vi "Set Pos Ctrl Paras.vi"(8 "error in (no error)":errorcluster, 10 "Pos Ctrl Paras":T1={"Tolerance(deg)"=0.5, "Loop Time(ms)"=10, "Min Frequency(hz)"=40.0} {"Min Frequency(hz)" format="%#_13g"}, 11 "SGDV_Ctrl_Class in":refnum<class "SGDV Motor.lvclass">) -> (0 "error out":errorcluster, 3 "SGDV_Ctrl_Class out":refnum<class "SGDV Motor.lvclass">)   [LabVIEW 2013, in "SGDV_Ctrl_v13_lib.lvlib" / "SGDV Motor.lvclass"]
uses:
  SGDV Motor.lvclass
  Controls and General VIs/Pos Ctrl Paras.ctl
  SGDV Motor.lvclass/SGDV Motor.ctl
  SGDV_Ctrl_v13_lib.lvlib
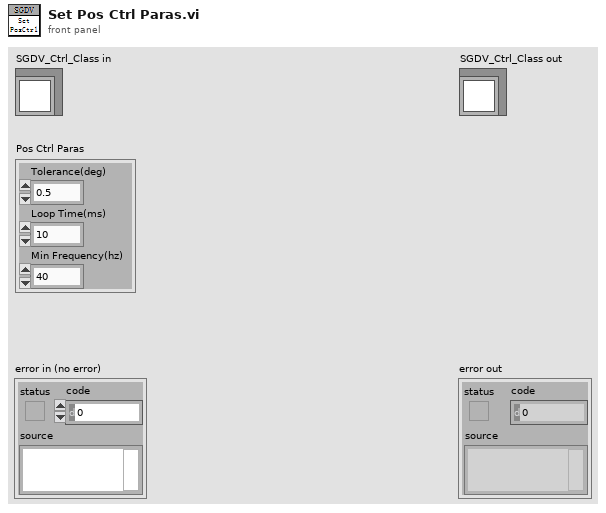
[diagram p1: front panel]
types:
  T1 = typedef "SGDV_Ctrl_v13_lib.lvlib/Pos Ctrl Paras.ctl" = cluster{"Tolerance(deg)":dbl, "Loop Time(ms)":u32, "Min Frequency(hz)":dbl}
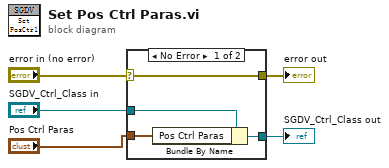
[diagram p0: block diagram]
diagram:
  n1 = case shown="No Error" "error in (no error)" {
    selector: "error in (no error)" -> [w9 w10]
    tunnel: [w9 w10] -> w4
    tunnel: [w7 w11] -> w2
    tunnel: "SGDV_Ctrl_Class in" -> [w8 w11]
    tunnel: "Pos Ctrl Paras" -> [w6 _]
    frame No Error {
      n2 = Bundle By Name(cluster=w8, "Pos Ctrl Paras"=w6) -> (w7:refnum<class "SGDV Motor.lvclass">)
    }
    frame Error {
    }
  }
  "error out" <- w4
  "SGDV_Ctrl_Class out" <- w2
